vi "Get Classes of Type.vi"(8 "error in (no error)":errorcluster, 10 "Class Type":refnum<class>, 11 "Directory Path":path) -> (0 "error out":errorcluster, 3 "Classes[]":refnum<class>[](array[class]))   [LabVIEW 2016, in "SLL Class.lvlib"]
doc: "Given a directory, get the list of classes (including those inside PPLs) which are of the given class type."
uses:
  SLL Class.lvlib
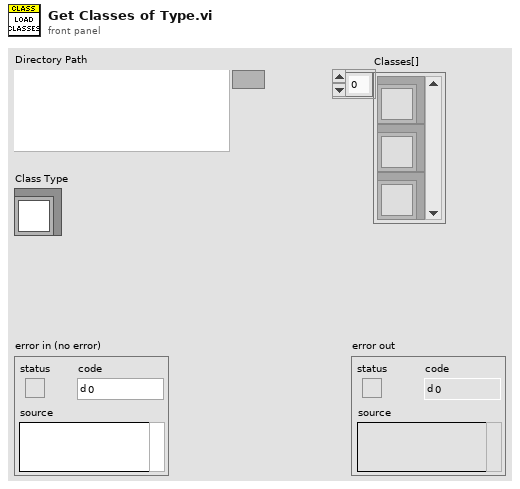
[diagram p1: front panel]
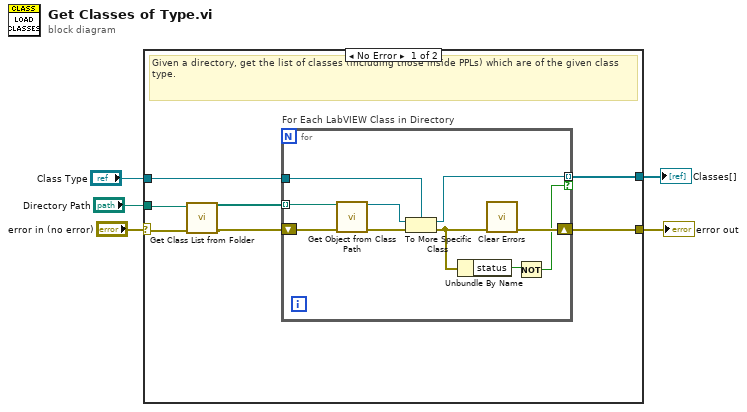
[diagram p0: block diagram]
diagram:
  n1 = case shown="No Error" "error in (no error)" {
    selector: "error in (no error)" -> [w10 w23]
    tunnel: [w12 w23] -> w4
    tunnel: "Directory Path" -> [w9 _]
    tunnel: "Class Type" -> [w11 _]
    tunnel: [w6 _] -> w1
    frame No Error {
      # "Given a directory, get the list of classes (including those inside PPLs) which are of the given class type."
      n2 = call "Get Class List from Folder.vi"("error in (no error)"=w10, "Folder Path"=w9) -> ("error out"=w7:errorcluster, "Class List[]"=w8:path[])  [unwired: 8 in]
      n3 = for "For Each LabVIEW Class in Directory" {
        shift-right: [w16] -> w12
        shift-left: w7 -> [w21]
        tunnel: w8 -> [w19] mode=indexing
        tunnel: w11 -> [w18]
        tunnel: [w17] -> w6 mode=indexing if=w13
        n4 = call "Get Object from Class Path.vi"("LabVIEW Class Path"=w19, "error in (no error)"=w21) -> ("Object"=w20:refnum<class>, "error out"=w22:errorcluster)  [unwired: 12 in]
        n5 = To More Specific Class(target class=w18, reference=w20, error in=w22) -> (specific class reference=w17:refnum<class>, error out=w15:errorcluster)
        n6 = Unbundle By Name(w15) -> ("status"=w14:bool)
        n7 = call <vilib>:"Clear Errors.vi"("error in (no error)"=w15) -> ("error out"=w16:errorcluster)  [unwired: 5 in, 1 out]
        n8 = Not(x=w14) -> (.not. x?=w13:bool)
      }
    }
    frame Error {
    }
  }
  "error out" <- w4
  "Classes[]" <- w1
